vi "Unflatten State.vi"(8 "error in":errorcluster, 10 "Flattened State":string) -> (0 "error out":errorcluster, 2 "State":T1)   [LabVIEW 2020, in "lv_icon.lvlib" / "History.lvlib"]
doc: "Unflattens the state so the individual parts of the state can be used."
uses:
  History.lvlib
  State.ctl
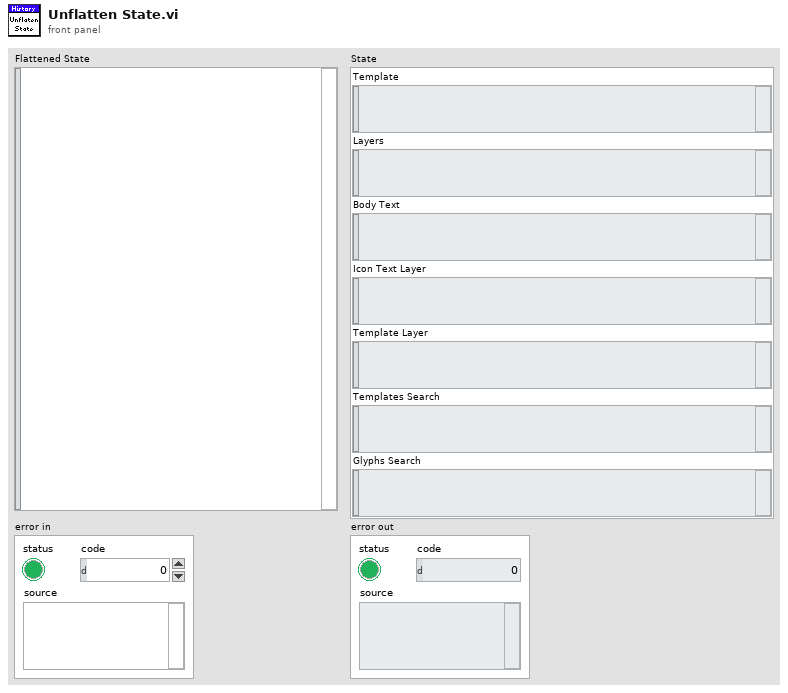
[diagram p1: front panel]
types:
  T1 = typedef "lv_icon.lvlib/History.lvlib/State.ctl" = cluster{"Template":string, "Layers":string, "Body Text":string, "Icon Text Layer":string, "Template Layer":string, "Templates Search":string, "Glyphs Search":string}
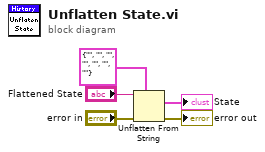
[diagram p0: block diagram]
diagram:
  n1 = Unflatten From String(type=T1 {"Template"="", "Layers"="", "Body Text"="", "Icon Text Layer"="", "Template Layer"="", "Templates Search"="", "Glyphs Search"=""} ("State"), binary string="Flattened State", error in (no error)="error in") -> (value=→"State":T1, error out=→"error out":errorcluster)  [unwired: 2 in, 1 out]
